vi "Set Table References.vi"(7 "Budget":refnum<vi>, 8 "error in (no error)":errorcluster, 9 "Credit":refnum<vi>, 10 "Banking":refnum<vi>, 11 "Budgetizer in":refnum<class "Budgetizer.lvclass">) -> (0 "error out":errorcluster, 3 "Budgetizer out":refnum<class "Budgetizer.lvclass">)   [LabVIEW 2018, in "Budgetizer.lvclass"]
uses:
  Budgetizer.lvclass
  Budgetizer.lvclass/Budgetizer.ctl
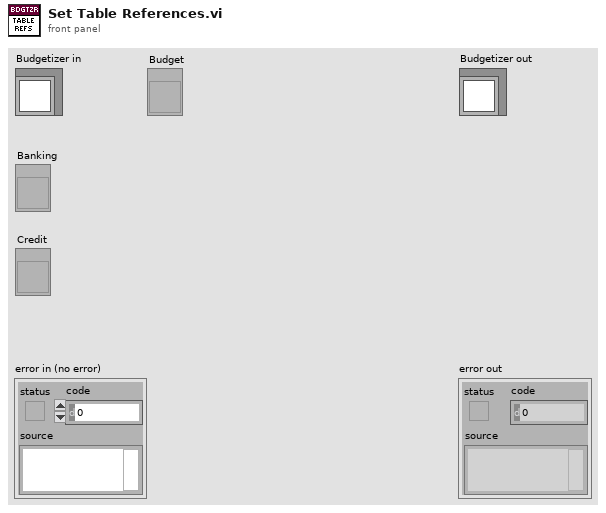
[diagram p1: front panel]
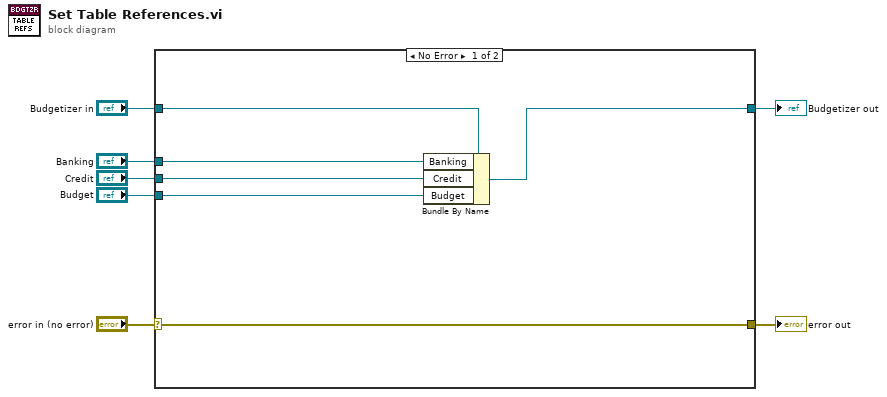
[diagram p0: block diagram]
diagram:
  n1 = case shown="No Error" "error in (no error)" {
    selector: "error in (no error)" -> [w13 w15]
    tunnel: [w13 w15] -> w6
    tunnel: [w11 w14] -> w4
    tunnel: "Budgetizer in" -> [w12 w14]
    tunnel: "Banking" -> [w10 _]
    tunnel: "Credit" -> [w9 _]
    tunnel: "Budget" -> [w8 _]
    frame No Error {
      n2 = Bundle By Name(cluster=w12, "Banking"=w10, "Credit"=w9, "Budget"=w8) -> (w11:refnum<class "Budgetizer.lvclass">)
    }
    frame Error {
    }
  }
  "error out" <- w6
  "Budgetizer out" <- w4
